vi "Check if Can Boost.vi"(11 "Flying Saucer in":refnum<class "Flying Saucer.lvclass">) -> (2 "Can Boost?":bool)   [LabVIEW 2021, in "Flying Saucer.lvclass"]
doc: "MIT Licence\nCopyright (c) 2024 David Grollier"
uses:
  Flying Saucer.lvclass
  Flying Saucer.lvclass/Flying Saucer.ctl
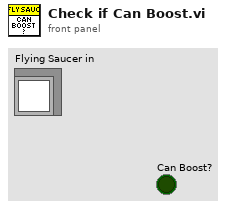
[diagram p1: front panel]
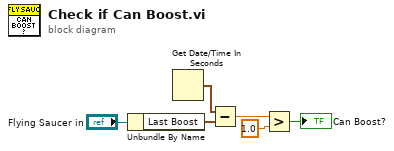
[diagram p0: block diagram]
diagram:
  n1 = Unbundle By Name("Flying Saucer in") -> ("Last Boost"=w4:timestamp)
  n2 = Get Date/Time In Seconds() -> (seconds since 1Jan1904=w5:timestamp)
  n3 = Subtract(x=w5, y=w4) -> (x-y=w3:dbl)
  n4 = Greater?(x=w3, y=1.0) -> (0:→"Can Boost?":bool)
